vi "kArrayBufferDbl.vi"(8 "HistLen":i32=100, 11 "Input Vect":dbl[](array[numeric])=[0.0, 0.0]) -> (3 "Output Array":dbl[][](array[numeric]))   [LabVIEW 2018, in "kevLib2010.lvlib"]
uses:
  kevLib2010.lvlib
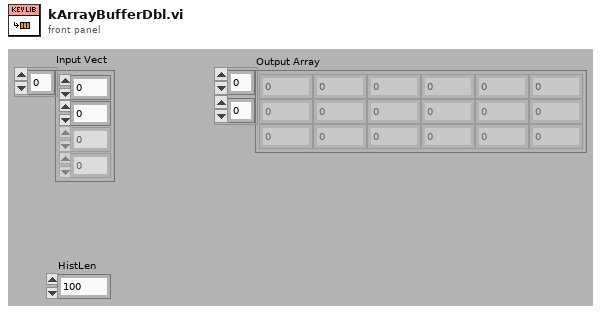
[diagram p1: front panel]
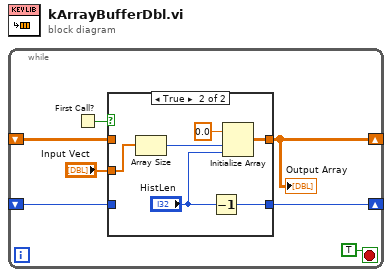
[diagram p0: block diagram]
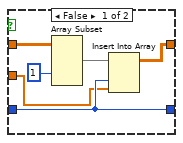
[diagram p2: hidden frame]
diagram:
  n1 = while {
    shift-right: [w2] -> _
    shift-left: _ -> [w5]
    shift-right: [w4] -> _
    shift-left: _ -> [w3]
    stop <- TRUE stop-if-true
    n2 = First Call?() -> (First Call?: T/F=w7:bool)
    n3 = case shown="True" w7 {
      tunnel: "Input Vect" -> [w8 w18]
      tunnel: [w11 w16] -> w2
      tunnel: w5 -> [w13 _]
      tunnel: [w9 w14] -> w4
      tunnel: w3 -> [w9 _]
      frame False {
        n4 = Array Subset(array=w13, index (col)=1 ("index")) -> (w12:dbl[][])  [unwired: 3 in]
        n5 = Insert Into Array(array=w12, index (col)=w9, new element=w8) -> (w11:dbl[][])  [unwired: 1 in]
      }
      frame True {
        n6 = Array Size(array=w18) -> (size(s)=w17:i32)
        n7 = Decrement(x="HistLen") -> (x-1=w14:i32)
        n8 = Initialize Array(0.0 ("element"), w17, "HistLen") -> (w16:dbl[][])
      }
    }
    "Output Array" <- w2
  }
